vi "MICSD Set Calibration Data.vi"(8 "error in (no error)":errorcluster, 9 "Calibration Data":u8[](array[numeric]) format="%02x", 10 "Register":enum16{"INFO_D", "INFO_C"}(ring), 11 "VISA Resource Name":refnum<visa-resource-name>) -> (0 "error out":errorcluster, 3 "dup VISA Resource Name":refnum<visa-resource-name>)   [LabVIEW 2020]
uses:
  <vilib>/Instr/_visa.llb/VISA Configure Serial Port (Instr).vi
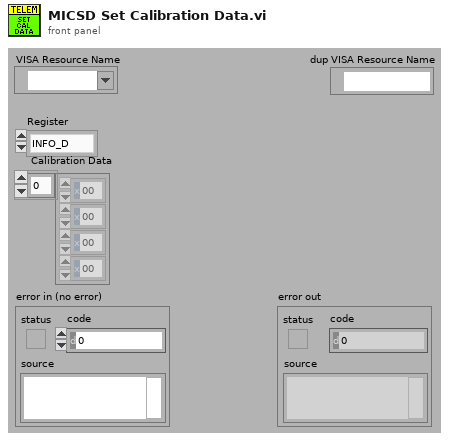
[diagram p1: front panel]
types:
  T1 = cluster{"Command Token":u8, "Length":u16, "Pack Data":u8[]}
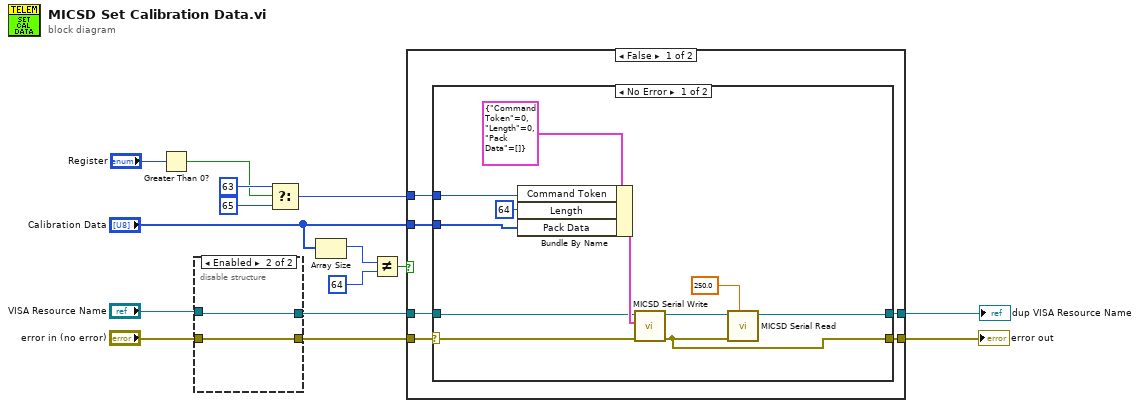
[diagram p0: block diagram]
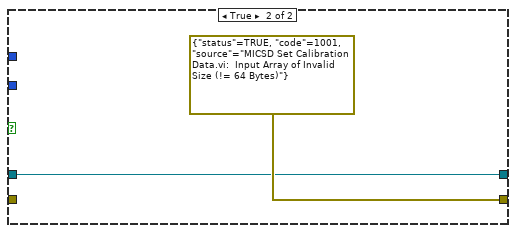
[diagram p3: hidden frame]
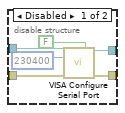
[diagram p4: hidden frame]
diagram:
  n1 = Greater Than 0?(x="Register") -> (x > 0?=w6:bool)
  n2 = disable-structure shown="Enabled" {
    disable-tunnel: [w19 w22] -> w14
    disable-tunnel: "error in (no error)" -> [w18 w22]
    disable-tunnel: "VISA Resource Name" -> [w17 w23]
    disable-tunnel: [w16 w23] -> w11
    frame Disabled {
      n3 = call-poly "VISA Configure Serial Port"("VISA resource name"=w17, "Enable Termination\nChar (T)"=FALSE ("Enable Termination\nChar (T)"), "baud rate (9600)"=u32 230400, "error in (no error)"=w18) -> ("VISA resource name out"=w16:refnum<visa-resource-name>, "error out"=w19:errorcluster)  [unwired: 10 in]
    }
    frame Enabled {
    }
  }
  n4 = Select(t=u16 63 ("Length"), s=w6, f=u16 65 ("Length")) -> (s? t:f=w9:u16)
  n5 = Array Size(array="Calibration Data") -> (size(s)=w3:i32)
  n6 = Not Equal?(x=w3, y=u16 64 ("Length")) -> (x != y?=w1:bool)
  n7 = case shown="False" w1 {
    tunnel: [w29 w43] -> w15
    tunnel: w14 -> [w28 _]
    tunnel: w11 -> [w27 w43]
    tunnel: [w26 errorcluster {"status"=TRUE, "code"=1001, "source"="MICSD Set Calibration Data.vi:  Input Array of Invalid Size (!= 64 Bytes)"} ("error IO")] -> w10
    tunnel: w9 -> [w25 _]
    tunnel: "Calibration Data" -> [w24 _]
    frame False {
      n8 = case shown="No Error" w28 {
        selector: w28 -> [w38 w42]
        tunnel: [w30 w42] -> w26
        tunnel: w27 -> [w37 w41]
        tunnel: [w31 w41] -> w29
        tunnel: w24 -> [w35 _]
        tunnel: w25 -> [w34 _]
        frame No Error {
          n9 = Bundle By Name(cluster=T1 {"Command Token"=0, "Length"=0, "Pack Data"=[]} ("Write Data"), "Command Token"=w34, "Length"=u16 64, "Pack Data"=w35) -> (w40:T1)
          n10 = call "MICSD Serial Write.vi"("error in (no error)"=w38, "Write Data"=w40, "VISA Resource Name"=w37) -> ("error out"=w30:errorcluster, "DUP Visa Resource Name"=w33:refnum<visa-resource-name>)  [unwired: 7 in]
          n11 = call "MICSD Serial Read.vi"("Timeout(mS)"=250.0, "error in (no error)"=w30, "VISA Resource Name"=w33) -> ("DUP Visa Resource Name"=w31:refnum<visa-resource-name>)  [unwired: 6 in, 2 out]
        }
        frame Error {
        }
      }
    }
    frame True {
    }
  }
  "dup VISA Resource Name" <- w15
  "error out" <- w10
